vi "DataLeveling.vi"(6 "거리 배열":dbl[](array[numeric]), 7 "LOG(AS)-LOG(S)":dbl[](array[numeric]), 8 "LOG(AS-S)":dbl[](array[numeric]), 9 "데이터 총량":u32) -> (0 "최종 거리 배열":dbl[](array[numeric]), 1 "LOG(AS)-LOG(S)":dbl[](array[numeric]), 2 "LOG(AS-S)":dbl[](array[numeric]), 3 "최종 데이터 수량":dbl)   [LabVIEW 2020]
uses:
  <vilib>/Analysis/6fits.llb/Curve Fitting Criteria.ctl
  <vilib>/Analysis/NI_AALPro.lvlib
panel:
  out "intercept":dbl caption="절편"
  out "slope":dbl caption="기울기"
  out "Best Linear Fit":dbl[](array[numeric]) caption="최적 선형 피팅"
  in  "필요평균수":dbl=20.0
  in  "제거할 데이터 끝점":dbl=700.0
  out "XY Graph":cluster{"Y":dbl[], "Y":dbl[]}[](graph) caption="XY 그래프"
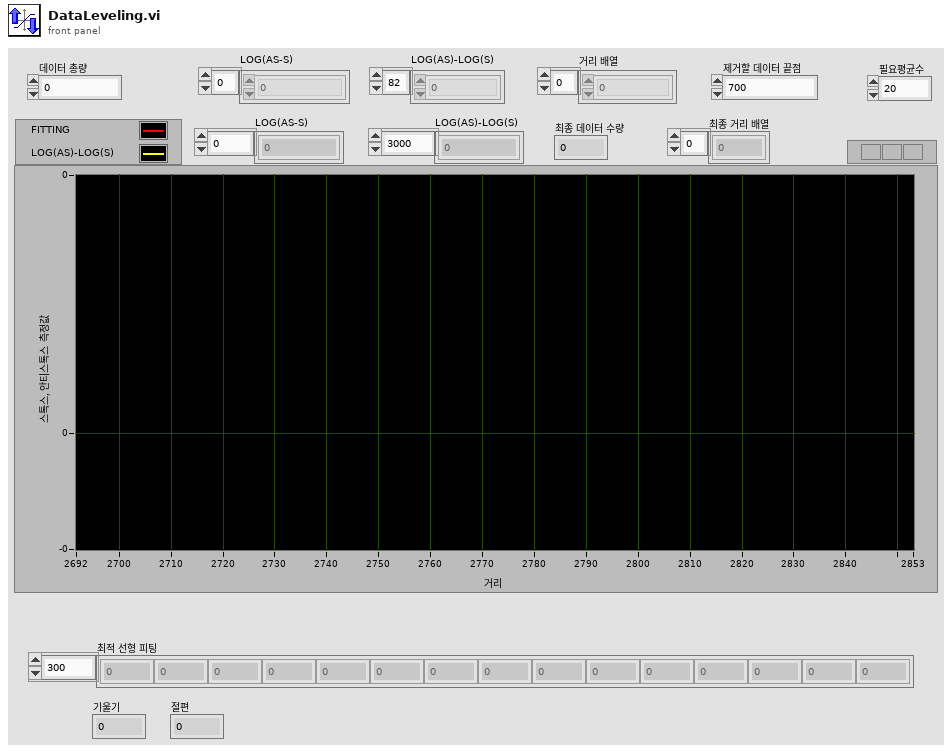
[diagram p1: front panel]
types:
  T1 = typedef "NI_AALPro.lvlib/Curve Fitting Criteria.ctl" = u16
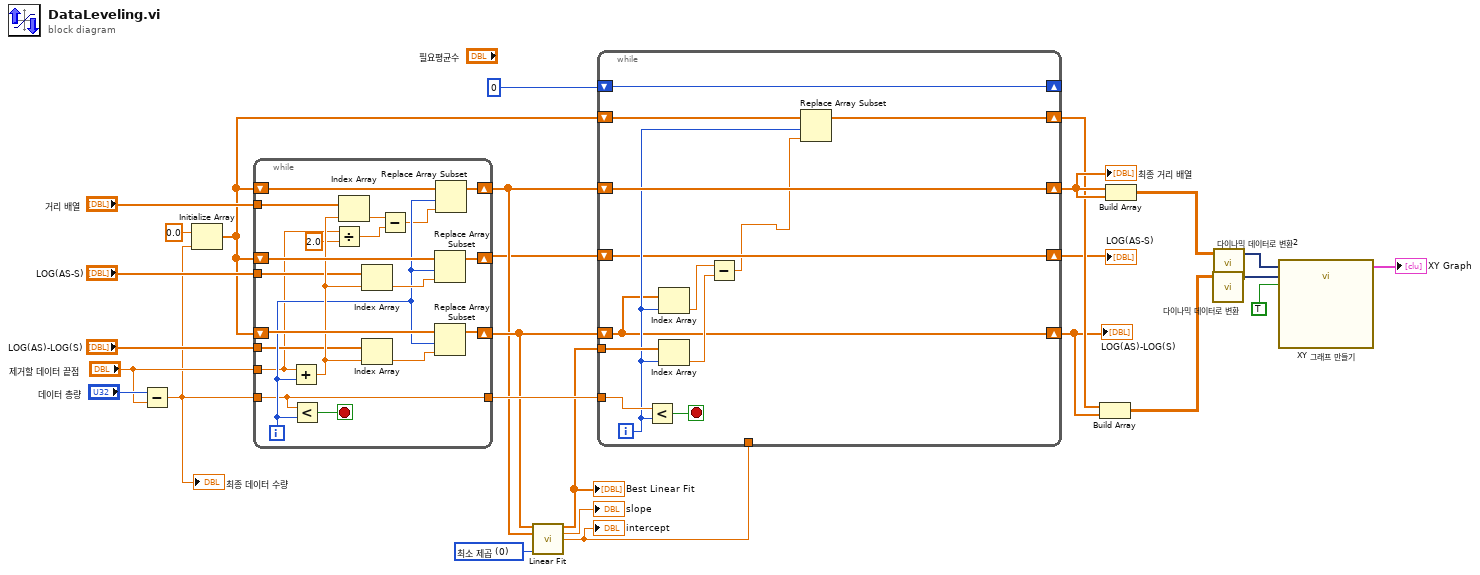
[diagram p0: block diagram]
diagram:
  w8 = T1 0 items=["최소 제곱", "최소 절대 오차", "바이스퀘어(Bisquare)"] ("method")
  n1 = Subtract(x="데이터 총량", y="제거할 데이터 끝점") -> (x-y=w14:dbl)
  "최종 데이터 수량" <- w14
  n2 = Initialize Array(0.0 ("원소"), w14) -> (w7:dbl[])
  n3 = while {
    tunnel: w14 -> [w28]
    shift-right: [w46] -> w4
    shift-left: w7 -> [w44]
    shift-right: [w45] -> w11
    shift-left: w7 -> [w43]
    tunnel: "제거할 데이터 끝점" -> [w29]
    shift-right: [w41] -> w9
    shift-left: w7 -> [w40]
    tunnel: "거리 배열" -> [w32]
    tunnel: "LOG(AS-S)" -> [w31]
    tunnel: "LOG(AS)-LOG(S)" -> [w30]
    tunnel: [w28] -> w13
    i -> [w38]
    stop <- w47 stop-if-true
    n4 = Add(x=w29, y=w38) -> (x+y=w39:dbl)
    n5 = Less?(x=w28, y=w38) -> (x < y?=w47:bool)
    n6 = Divide(x=w29, y=2.0) -> (x/y=w34:dbl)
    n7 = Index Array(array=w32, index=w39) -> (element=w36:dbl)
    n8 = Index Array(array=w31, index=w39) -> (element=w42:dbl)
    n9 = Index Array(array=w30, index=w39) -> (element=w37:dbl)
    n10 = Subtract(x=w36, y=w34) -> (x-y=w35:dbl)
    n11 = Replace Array Subset(array=w44, new element=w42, index=w38) -> (w46:dbl[])
    n12 = Replace Array Subset(array=w43, new element=w37, index=w38) -> (w45:dbl[])
    n13 = Replace Array Subset(array=w40, new element=w35, index=w38) -> (w41:dbl[])
  }
  n14 = call <vilib>:"Linear Fit.vi"("Y"=w11, "X"=w9, "method"=w8) -> ("Best Linear Fit"=w6:dbl[], "slope"=→"slope":dbl, "intercept"=w1:dbl)  [unwired: 8 in, 2 out]
  "Best Linear Fit" <- w6
  "intercept" <- w1
  n15 = while {
    shift-right: [w57] -> w15
    shift-left: w9 -> [w57]
    shift-right: [w49] -> w2
    shift-left: w11 -> [w49]
    tunnel: w13 -> [w59]
    shift-right: [w58] -> _
    shift-left: 0 -> [w58]
    shift-right: [w51] -> w5
    shift-left: w7 -> [w53]
    tunnel: w6 -> [w56]
    shift-right: [w50] -> w3
    shift-left: w4 -> [w50]
    tunnel: w1 -> [_]
    i -> [w52]
    stop <- w60 stop-if-true
    n16 = Less?(x=w59, y=w52) -> (x < y?=w60:bool)
    n17 = Index Array(array=w49, index=w52) -> (element=w55:dbl)
    n18 = Index Array(array=w56, index=w52) -> (element=w54:dbl)
    n19 = Subtract(x=w55, y=w54) -> (x-y=w48:dbl)
    n20 = Replace Array Subset(array=w53, new element=w48, index=w52) -> (w51:dbl[])
  }
  "LOG(AS-S)" <- w3
  "LOG(AS)-LOG(S)" <- w2
  "최종 거리 배열" <- w15
  n21 = Build Array(w5, w2) -> (w23:dbl[][])
  n22 = Build Array(w15, w15) -> (w22:dbl[][])
  n23 = call "다이나믹 데이터로 변환"("2D Array"=w23) -> ("Dynamic Data Type"=w25:dynamicdata)  [unwired: 3 in]
  n24 = call "다이나믹 데이터로 변환2"("2D Array"=w22) -> ("Dynamic Data Type"=w26:dynamicdata)  [unwired: 3 in]
  n25 = call "XY 그래프 만들기"("Reset"=TRUE, "Y Input"=w25, "X Input"=w26) -> ("XY Graph"=→"XY Graph":cluster{"X":dbl[], "Y":dbl[]}[])  [unwired: 7 in, 1 out]
